vi "Parse Message Default.vi"(7 "path":string[](array[string])=["message"], 8 "error in (no error)":errorcluster, 10 "content.@type":string, 11 "JSON (UTF-8) String":string) -> (0 "error out":errorcluster, 3 "New Message Text":T1)   [LabVIEW 2015, in "JSON Library.lvlib"]
doc: "Created IvanLis by LabVIEW Portal\nProfile: http://labviewportal.org/memberlist.php?mode=viewprofile&u=987\neMail: IvanLisanov@gMail.com\nTelegram: https://t.me/IvanLis"
uses:
  JSON Library.lvlib
  TypeDef/Message Text.ctl
  TypeDef/Message Default.ctl
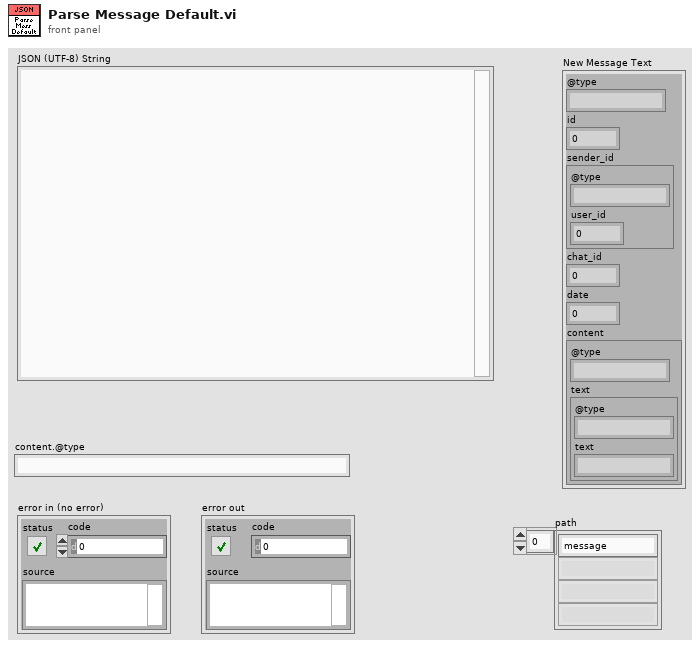
[diagram p1: front panel]
types:
  T1 = typedef "JSON Library.lvlib/Message Text.ctl" = cluster{"@type":string, "id":i64, "sender_id":cluster{"@type":string, "user_id":i64}, "chat_id":i64, "date":i64, "content":cluster{"@type":string, "text":cluster{"@type":string, "text":string}}}
  T2 = typedef "JSON Library.lvlib/Message Default.ctl" = cluster{"@type":string, "id":i64, "sender_id":cluster{"@type":string, "user_id":i64}, "chat_id":i64, "date":i64, "content":cluster{"@type":string}}
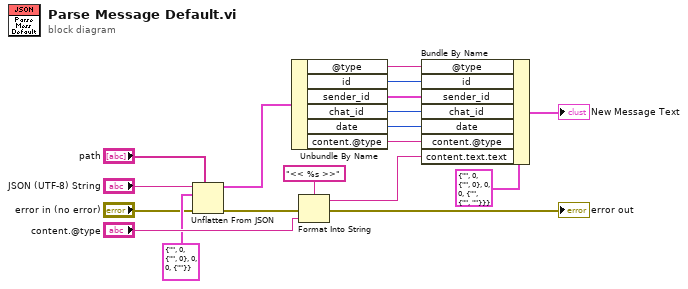
[diagram p0: block diagram]
diagram:
  n1 = Unflatten From JSON(path="path", JSON string="JSON (UTF-8) String", type and defaults=T2 {"@type"="", "id"=0, "sender_id"={"@type"="", "user_id"=0}, "chat_id"=0, "date"=0, "content"={"@type"=""}} ("Message Text"), error in (no error)="error in (no error)") -> (value=w6:T2, error out=w14:errorcluster)  [unwired: 3 in]
  n2 = Unbundle By Name(w6) -> ("@type"=w7:string, "id"=w8:i64, "sender_id"=w9:cluster{"@type":string, "user_id":i64}, "chat_id"=w10:i64, "date"=w11:i64, "content.@type"=w12:string)
  n3 = Format Into String(format string="<< %s >>", error in=w14, "content.@type") -> (resulting string=w13:string, error out=→"error out":errorcluster)  [unwired: 1 in]
  n4 = Bundle By Name(cluster=T1 {"@type"="", "id"=0, "sender_id"={"@type"="", "user_id"=0}, "chat_id"=0, "date"=0, "content"={"@type"="", "text"={"@type"="", "text"=""}}} ("New Message Text"), "@type"=w7, "id"=w8, "sender_id"=w9, "chat_id"=w10, "date"=w11, "content.@type"=w12, "content.text.text"=w13) -> (→"New Message Text":T1)
